vi "Create Event.vi"(8 "error in (no error)":errorcluster, 11 "OnChange_Boolean in":refnum<class "OnChangeNotifier_Varient.lvclass">) -> (0 "error out":errorcluster, 3 "OnChange_Boolean out":refnum<class "OnChangeNotifier_Varient.lvclass">)   [LabVIEW 2021, in "OnChangeNotifier_Varient.lvclass"]
uses:
  OnChangeNotifier_Varient.lvclass
  OnChangeNotifier_Varient.lvclass/OnChangeNotifier_Varient.ctl
  Support/Type.ctl
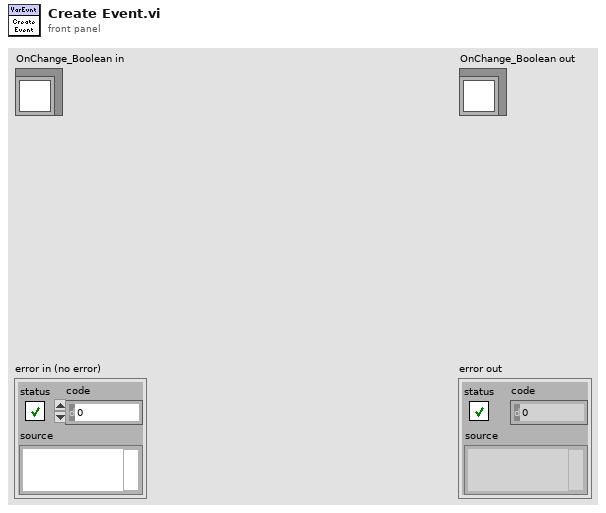
[diagram p1: front panel]
types:
  T1 = typedef "OnChangeNotifier_Varient.lvclass/Type.ctl" = variant
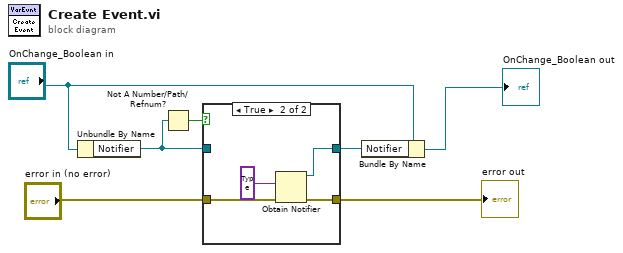
[diagram p0: block diagram]
diagram:
  n1 = Unbundle By Name("OnChange_Boolean in") -> ("Notifier"=w1:refnum<notifier>)
  n2 = Not A Number/Path/Refnum?(number/path/refnum=w1) -> (NaN/Path/Refnum?=w2:bool)
  n3 = case shown="True" w2 {
    tunnel: "error in (no error)" -> [w8 w13]
    tunnel: [w9 w12] -> w5
    tunnel: [w8 w10] -> w4
    tunnel: w1 -> [w9 _]
    frame False {
    }
    frame True {
      n4 = Obtain Notifier(notification data type=T1 variant(u8 0) ("Value"), error in (no error)=w13) -> (notifier out=w12:refnum<notifier>, error out=w10:errorcluster)  [unwired: 2 in, 1 out]
    }
  }
  "error out" <- w4
  n5 = Bundle By Name(cluster="OnChange_Boolean in", "Notifier"=w5) -> (→"OnChange_Boolean out":refnum<class "OnChangeNotifier_Varient.lvclass">)
